vi "PWMControl.vi"() -> ()   [LabVIEW 2016]
uses:
  <vilib>/Utility/error.llb/DialogType.ctl
  <vilib>/DAQmx/write.llb/DAQmx Write (Digital 1D Bool 1Chan 1Samp).vi
  <vilib>/DAQmx/read.llb/DAQmx Read (Analog 1D Wfm NChan NSamp).vi
  <vilib>/DAQmx/configure/task.llb/DAQmx Configure Logging (TDMS).vi
  <vilib>/DAQmx/configure/timing.llb/DAQmx Timing (Sample Clock).vi
  <vilib>/DAQmx/create/channels.llb/DAQmx Create Channel (DO-Digital Output).vi
  <vilib>/DAQmx/miscellaneous.llb/DAQmx Fill In Error Info.vi
  <resource>/objmgr/daqmx.rc
panel:
  in  "Lines":tag="Dev1/port0/line0:7" caption="Digital output line"
  in  "Idle State 2":bool
  in  "Duty cycle % (0-100) 2":dbl=50.0
  in  "Cycle time PWM (seconds) 2":i32=5
  in  "Steps in a cycle 2":i32=256
  out "Output 2":i16(graph)
  in  "base path":path=path "C:/Users/mmunoz/Desktop/Summer Coding Files/Labview Practice Codes/Compiled Data files"
  out "error out":errorcluster
  in  "error in":errorcluster
  in  "Show Configure Dialog?":bool
  in  "Remove Extra Properties? (T)":bool=TRUE
  in  "File Name":string="junk"
  in  "stop 2":bool
  out "Time Elapsed":dbl format="%<%H:%M:%S%2u>t"
  out "Waveform Chart":waveform(dbl)[](graph)
  out "DAQ error":string
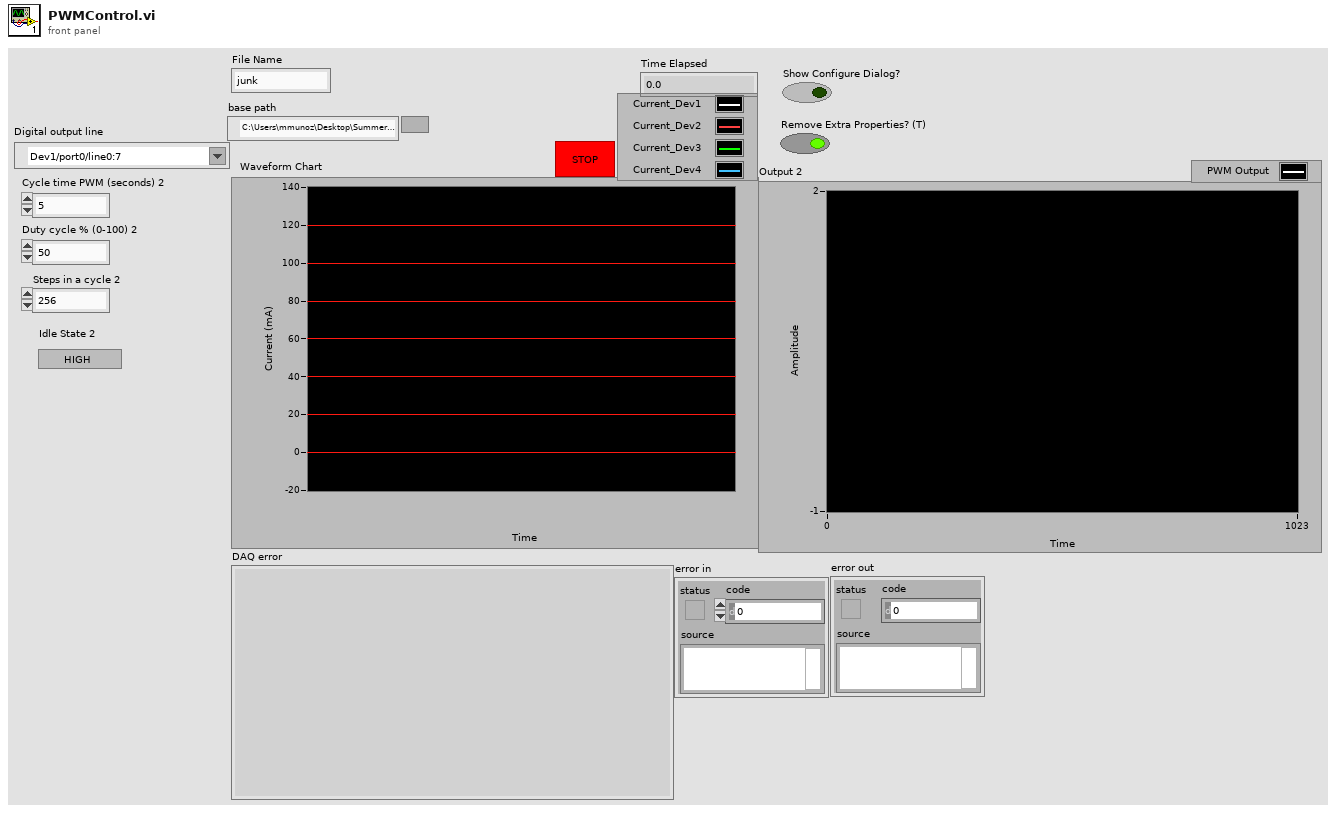
[diagram p1: front panel]
types:
  T1 = typedef "DialogType.ctl" = u16
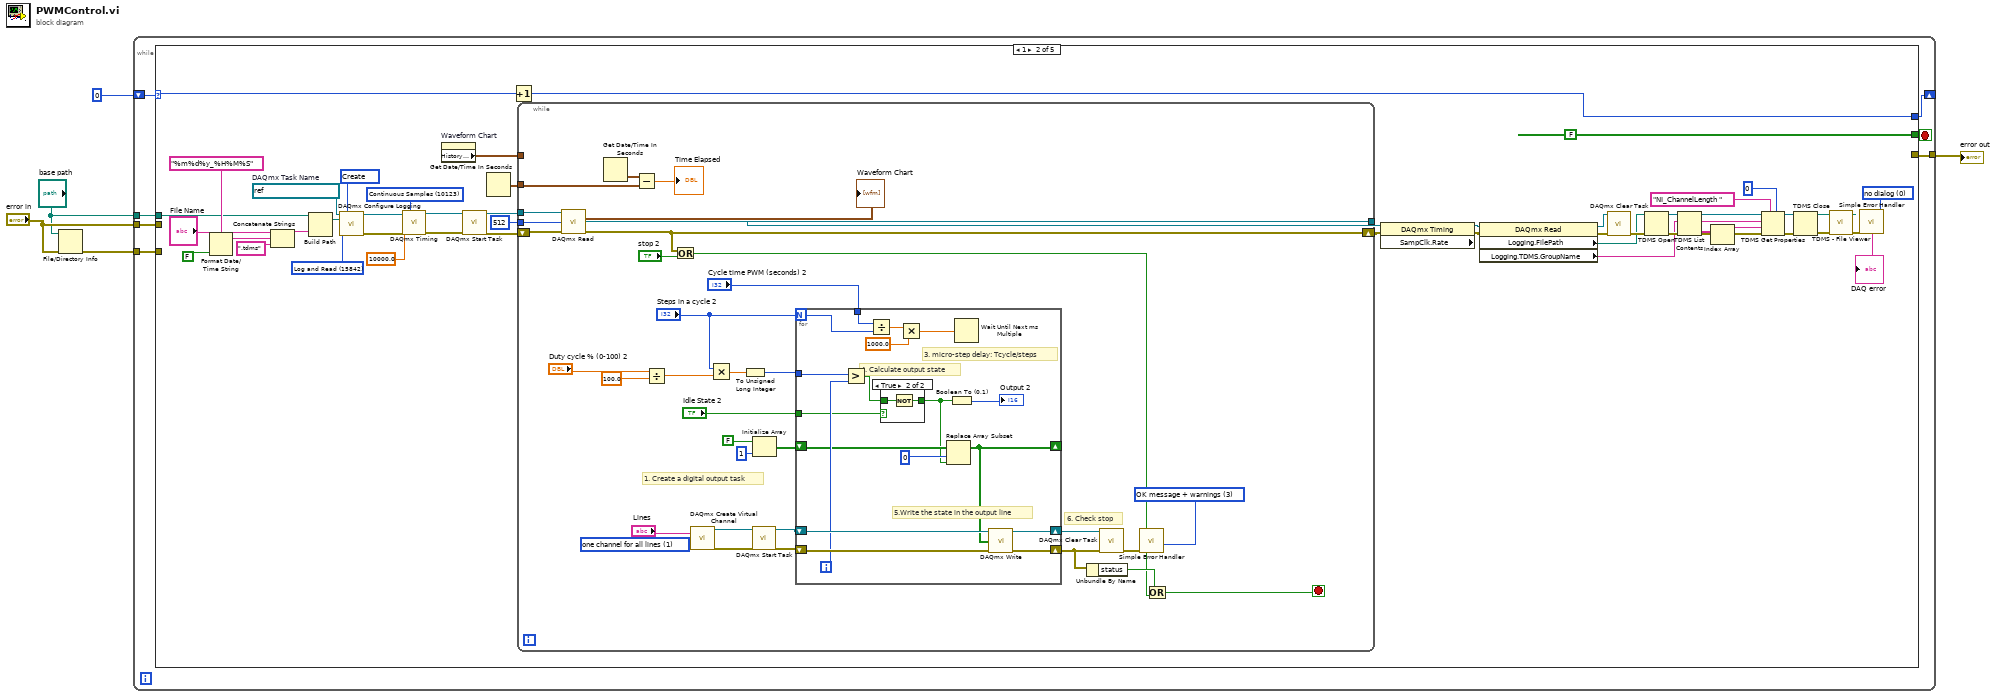
[diagram p0: block diagram]
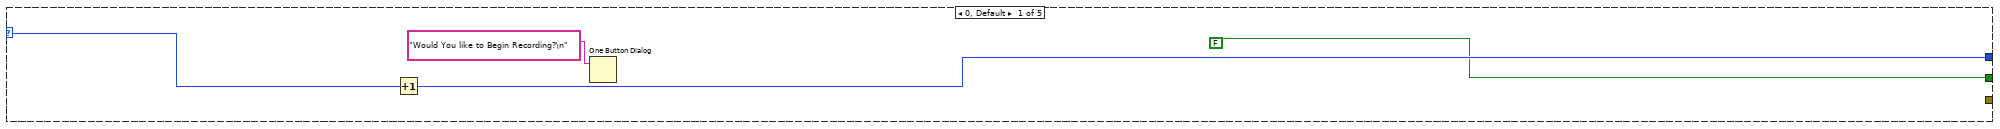
[diagram p2: hidden frame]
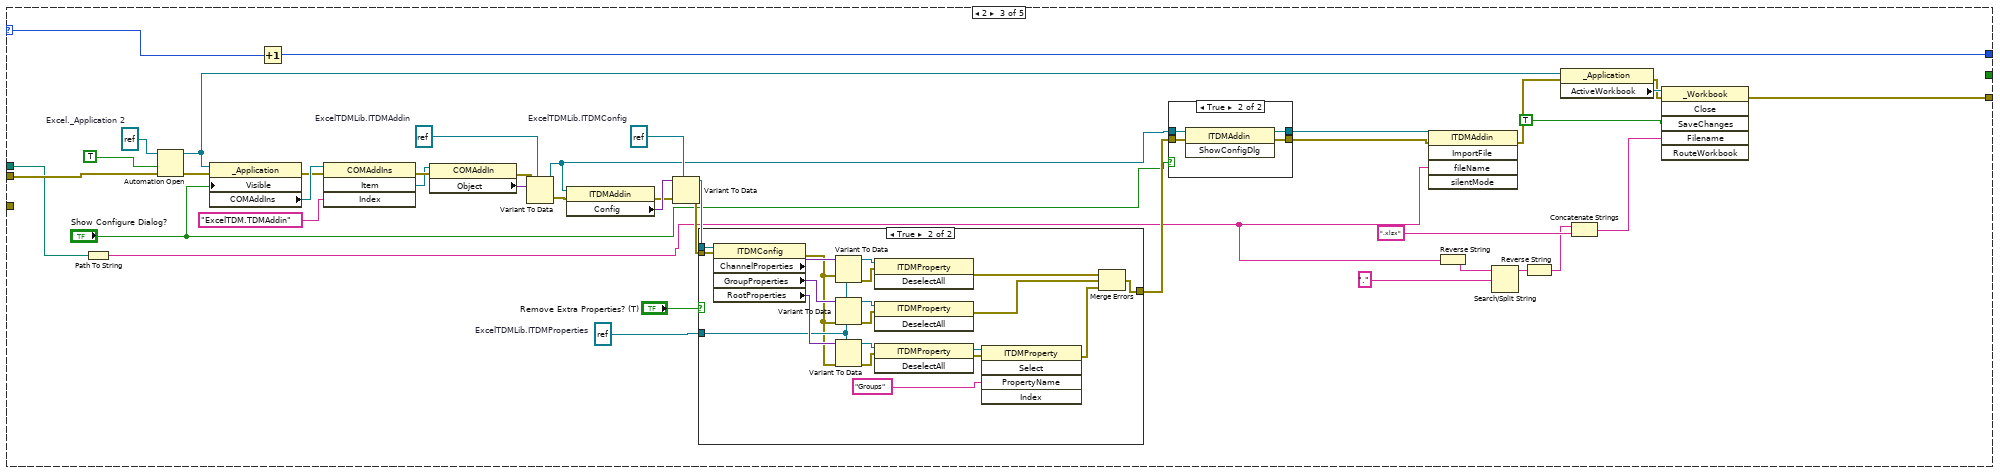
[diagram p4: hidden frame]
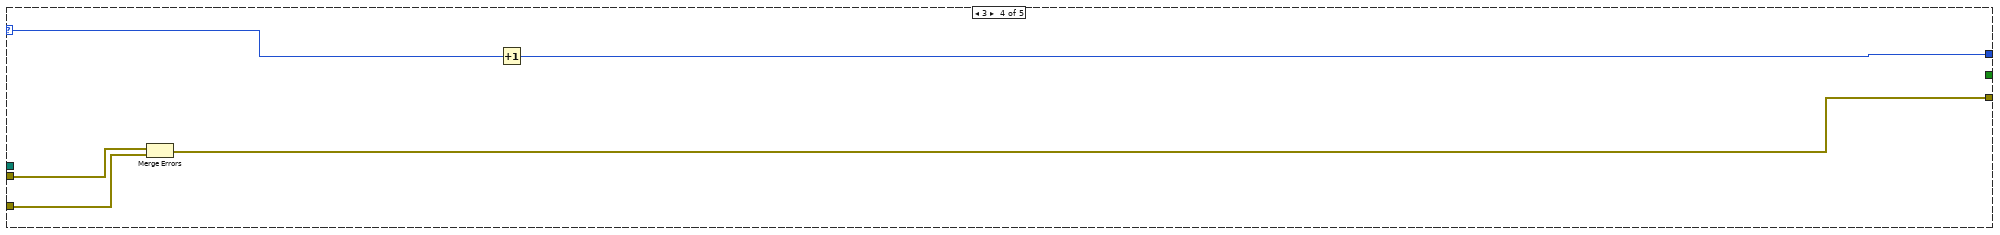
[diagram p7: hidden frame]
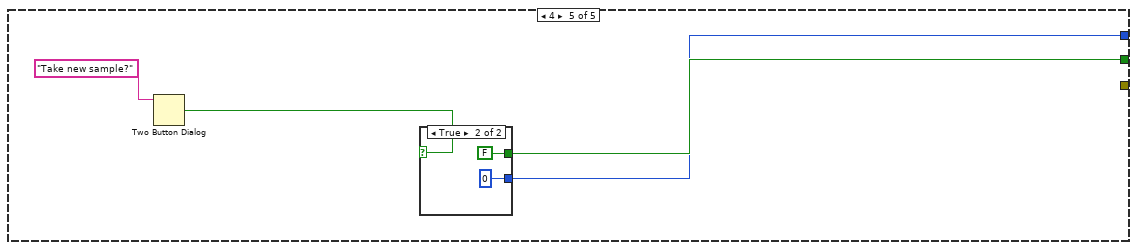
[diagram p8: hidden frame]
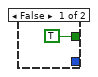
[diagram p9: hidden frame]
diagram:
  n1 = File/Directory Info(path="base path", error in="error in") -> (error out=w3:errorcluster)  [unwired: 6 out]
  n2 = while {
    shift-right: [w11] -> _
    shift-left: 0 -> [w12]
    tunnel: "error in" -> [w10]
    tunnel: w3 -> [w9]
    tunnel: [w8] -> w2
    tunnel: "base path" -> [w7]
    stop <- w6 stop-if-true
    n3 = case shown="1" w12 {
      selector: w12 -> [w13 w44 w162 w191 _]
      tunnel: [w15 w43 w161 w190 w195] -> w11
      tunnel: [FALSE FALSE _ _ w196] -> w6
      tunnel: w10 -> [_ _ w149 w193 _]
      tunnel: w9 -> [_ _ _ w194 _]
      tunnel: [_ _ w128 w192 _] -> w8
      tunnel: w7 -> [_ w17 w122 _ _]
      frame 0, Default {
        n4 = Increment(x=w13) -> (x+1=w15:i32)
        n5 = One Button Dialog(message="Would You like to Begin Recording?\n" ("initial string")) -> ()  [unwired: 1 in, 1 out]
      }
      frame 1 {
        w25 = 10123 items=["Finite Samples"=10178, "Continuous Samples"=10123, "Hardware Timed Single Point"=12522] ("sample mode")
        w52 = T1 0 items=["no dialog", "OK message", "continue or stop message", "OK message + warnings", "continue/stop + warnings"] ("type of dialog (OK msg:1)")
        w57 = 15848 items=["Open"=10437, "Open or Create"=15846, "Create or Replace"=15847, "Create"=15848] ("operation")
        w59 = 15842 items=["Off"=10231, "Log"=15844, "Log and Read"=15842] ("logging mode")
        w60 = refnum<k21> "DAQ Assistant_0"  # DAQmx Task Name
        n6 = Format Date/Time String(time format string (%c)="%m%d%y_%H%M%S", UTC format=FALSE) -> (date/time string=w63:string)  [unwired: 1 in]
        n7 = Concatenate Strings("File Name", w63, ".tdms") -> (w64:string)
        n8 = Build Path(base path=w17, name or relative path=w64) -> (appended path=w58:path)
        n9 = call-poly <vilib>:"DAQmx Configure Logging.vi"("task/channels in"=w60, "operation"=w57, "file path"=w58, "logging mode"=w59) -> ("task out"=w26:refnum<k21>, "error out"=w27:errorcluster)  [unwired: 10 in]
        n10 = call-poly <vilib>:"DAQmx Timing.vi"("task/channels in"=w26, "sample mode"=w25, "rate"=10000.0, "error in"=w27) -> ("task out"=w24:refnum<k21>, "error out"=w23:errorcluster)  [unwired: 10 in]
        n11 = property on="Waveform Chart" class="WFChart (strict)"() -> ("History Data"=w21:waveform(dbl)[][])  [unwired: 2 in, 2 out]
        n12 = call <vilib>:"DAQmx Start Task.vi"("task/channels in"=w24, "error in"=w23) -> ("task out"=w55:refnum<k21>, "error out"=w56:errorcluster)  [unwired: 12 in]
        n13 = Get Date/Time In Seconds() -> (seconds since 1Jan1904=w42:timestamp)
        n14 = Increment(x=w44) -> (x+1=w43:i32)
        n15 = while {
          tunnel: [w99] -> w31
          shift-right: [w92] -> w30
          shift-left: w56 -> [w98]
          tunnel: 512 -> [w97]
          tunnel: w55 -> [w96]
          tunnel: w42 -> [w95]
          tunnel: w21 -> [_]
          stop <- w67 stop-if-true
          w72 = T1 3 items=["no dialog", "OK message", "continue or stop message", "OK message + warnings", "continue/stop + warnings"] ("type of dialog (OK msg:1)")
          w78 = 1 items=["one channel for each line", "one channel for all lines"] ("line grouping")
          # "1. Create a digital output task"
          # "6. Check stop"
          n16 = call-poly <vilib>:"DAQmx Read.vi"("task/channels in"=w96, "number of samples per channel"=w97, "error in"=w98) -> ("task out"=w99:refnum<k21>, "data"=→"Waveform Chart":waveform(dbl)[], "error out"=w92:errorcluster)  [unwired: 10 in]
          n17 = Get Date/Time In Seconds() -> (seconds since 1Jan1904=w94:timestamp)
          n18 = Subtract(x=w94, y=w95) -> (x-y=→"Time Elapsed":dbl)
          n19 = Divide(x="Duty cycle % (0-100) 2", y=100.0) -> (x/y=w87:dbl)
          n20 = Or(x=w92, y="stop 2") -> (x .or. y?=w68:bool)
          n21 = call-poly <vilib>:"DAQmx Create Virtual Channel.vi"("lines"="Lines", "line grouping"=w78) -> ("task out"=w75:refnum<k21>, "error out"=w76:errorcluster)  [unwired: 12 in]
          n22 = Multiply(x="Steps in a cycle 2", y=w87) -> (x*y=w82:dbl)
          n23 = To Unsigned Long Integer(number=w82) -> (unsigned 32bit integer=w81:u32)
          n24 = call <vilib>:"DAQmx Start Task.vi"("task/channels in"=w75, "error in"=w76) -> ("task out"=w74:refnum<k21>, "error out"=w73:errorcluster)  [unwired: 12 in]
          n25 = Initialize Array(FALSE, 1 ("dimension size")) -> (w84:bool[])
          n26 = for {
            N: "Steps in a cycle 2" -> [w117]
            tunnel: "Cycle time PWM (seconds) 2" -> [w118]
            tunnel: w81 -> [w114]
            shift-right: [w113] -> w71
            shift-left: w74 -> [w110]
            shift-right: [w112] -> w70
            shift-left: w73 -> [w111]
            shift-right: [w105] -> _
            shift-left: w84 -> [w106]
            tunnel: "Idle State 2" -> [w104]
            i -> [w107]
            # "5.Write the state in the output line"
            # "4. Calculate output state"
            # "3. micro-step delay: Tcycle/steps"
            n27 = Greater?(x=w114, y=w107) -> (0:w103:bool)
            n28 = Divide(x=w118, y=w117) -> (x/y=w116:dbl)
            n29 = case shown="True" w104 {
              tunnel: [w119 w120] -> w102
              tunnel: w103 -> [w119 w121]
              frame False {
              }
              frame True {
                n30 = Not(x=w121) -> (.not. x?=w120:bool)
              }
            }
            n31 = Multiply(x=w116, y=1000.0) -> (x*y=w109:dbl)
            n32 = Replace Array Subset(array=w106, new element=w102, index=0) -> (w105:bool[])
            n33 = Boolean To (0,1)(Boolean=w102) -> (0, 1=→"Output 2":i16)
            n34 = Wait Until Next ms Multiple(millisecond multiple=w109) -> ()  [unwired: 1 out]
            n35 = call-poly <vilib>:"DAQmx Write.vi"("task/channels in"=w110, "data"=w105, "error in"=w111) -> ("task out"=w113:refnum<k21>, "error out"=w112:errorcluster)  [unwired: 10 in, 1 out]
          }
          n36 = Unbundle By Name(w70) -> ("status"=w79:bool)
          n37 = call <vilib>:"DAQmx Clear Task.vi"("task in"=w71, "error in"=w70) -> ("error out"=w69:errorcluster)  [unwired: 13 in]
          n38 = call <vilib>:"Simple Error Handler.vi"("type of dialog (OK msg:1)"=w72, "error in (no error)"=w69) -> ()  [unwired: 3 in, 5 out]
          n39 = Or(x=w79, y=w68) -> (x .or. y?=w67:bool)
        }
        n40 = property on="Property Node" class="DAQmx Timing" props=["SampClk.Rate"](reference=w31, error in=w30) -> (reference out=w29:refnum<k21>, error out=w28:errorcluster)  [unwired: 1 out]
        n41 = property on="Property Node" class="DAQmx Read"(reference=w29, error in=w28) -> (reference out=w51:refnum<k21>, error out=w50:errorcluster, "Logging.FilePath"=w45:path, "Logging.TDMS.GroupName"=w39:string)
        n42 = call <vilib>:"DAQmx Clear Task.vi"("task in"=w51, "error in"=w50) -> ("error out"=w46:errorcluster)  [unwired: 13 in]
        n43 = TDMS Open(8:w46, 11:w45) -> (0:w40:errorcluster, 3:w38:refnum<k34>)  [unwired: 5 in]
        n44 = TDMS List Contents(4:w40, 6:w39, 7:w38) -> (0:w18:errorcluster, 1:w36:string[], 2:w37:string, 3:w33:refnum<k34>)
        n45 = Index Array(array=w36) -> (element=w35:string)  [unwired: 1 in]
        n46 = TDMS Get Properties(5:0, 7:"NI_ChannelLength " ("property name"), 8:w18, 9:w35, 10:w37, 11:w33) -> (0:w19:errorcluster, 3:w20:refnum<k34>)  [unwired: 4 out]
        n47 = TDMS Close(8:w19, 11:w20) -> (0:w48:errorcluster, 3:w47:path)
        n48 = call <vilib>:"TDMS - File Viewer.vi"("error in (no error)"=w48, "file path"=w47) -> ("error out"=w49:errorcluster)  [unwired: 4 in, 1 out]
        n49 = call <vilib>:"Simple Error Handler.vi"("error code (no error:0)"=w52, "error in (no error)"=w49) -> ("message"=→"DAQ error":string)  [unwired: 3 in, 4 out]
      }
      frame 2 {
        w147 = refnum<k7> refnum  # ExcelTDMLib.ITDMProperties
        w158 = refnum<k7> refnum  # Excel._Application 2
        w154 = refnum<k7> refnum  # ExcelTDMLib.ITDMConfig
        w159 = refnum<k7> refnum  # ExcelTDMLib.ITDMAddin
        n50 = Path To String(path=w122) -> (string=w129:string)
        n51 = Automation Open(error in (no error)=w149, Automation Refnum=w158, 9:TRUE ("open new instance (false)")) -> (Automation Refnum=w127:refnum<k7>, error out=w157:errorcluster)  [unwired: 1 in]
        n52 = property class="_Application"(reference=w127, error in=w157, "Visible"="Show Configure Dialog?") -> (error out=w155:errorcluster, "COMAddIns"=w160:refnum<k7>)  [unwired: 1 out]
        n53 = Increment(x=w162) -> (x+1=w161:i32)
        n54 = invoke class="COMAddIns" method="Item"(reference=w160, error in=w155, "Index"="ExcelTDM.TDMAddin") -> (error out=w126:errorcluster, "Item"=w125:refnum<k7>)  [unwired: 1 in, 2 out]
        n55 = property class="COMAddIn"(reference=w125, error in=w126) -> (error out=w123:errorcluster, "Object"=w124:variant)  [unwired: 1 out]
        n56 = Variant To Data(error in=w123, type=w159, Variant=w124) -> (data=w143:refnum<k7>, error out=w152:errorcluster)
        n57 = property class="ITDMAddin"(reference=w143, error in=w152) -> (error out=w151:errorcluster, "Config"=w153:variant)  [unwired: 1 out]
        n58 = Variant To Data(error in=w151, type=w154, Variant=w153) -> (data=w144:refnum<k7>, error out=w145:errorcluster)
        n59 = case shown="True" "Remove Extra Properties? (T)" {
          tunnel: w147 -> [_ w185]
          tunnel: w145 -> [w169 w176]
          tunnel: w144 -> [_ w175]
          tunnel: [w169 w174] -> w146
          frame False {
          }
          frame True {
            n60 = property class="ITDMConfig"(reference=w175, error in=w176) -> (error out=w180:errorcluster, "ChannelProperties"=w189:variant, "GroupProperties"=w187:variant, "RootProperties"=w186:variant)  [unwired: 1 out]
            n61 = Variant To Data(error in=w180, type=w185, Variant=w189) -> (data=w188:refnum<k7>, error out=w177:errorcluster)
            n62 = Variant To Data(error in=w180, type=w185, Variant=w187) -> (data=w183:refnum<k7>, error out=w178:errorcluster)
            n63 = Variant To Data(error in=w180, type=w185, Variant=w186) -> (data=w184:refnum<k7>, error out=w179:errorcluster)
            n64 = invoke class="ITDMProperty" method="DeselectAll"(reference=w188, error in=w177) -> (error out=w181:errorcluster)  [unwired: 1 in, 2 out]
            n65 = invoke class="ITDMProperty" method="DeselectAll"(reference=w183, error in=w178) -> (error out=w182:errorcluster)  [unwired: 1 in, 2 out]
            n66 = invoke class="ITDMProperty" method="DeselectAll"(reference=w184, error in=w179) -> (reference out=w173:refnum<k7>, error out=w172:errorcluster)  [unwired: 1 in, 1 out]
            n67 = invoke class="ITDMProperty" method="Select"(reference=w173, error in=w172, "PropertyName"="Groups" ("string")) -> (error out=w171:errorcluster)  [unwired: 2 in, 4 out]
            n68 = Merge Errors(w181, w182, w171) -> (w174:errorcluster)
          }
        }
        n69 = case shown="True" "Show Configure Dialog?" {
          tunnel: w143 -> [w164 w168]
          tunnel: w146 -> [w163 w167]
          tunnel: [w163 w166] -> w130
          tunnel: [w164 w165] -> w131
          frame False {
          }
          frame True {
            n70 = invoke class="ITDMAddin" method="ShowConfigDlg"(reference=w168, error in=w167) -> (reference out=w165:refnum<k7>, error out=w166:errorcluster)  [unwired: 1 in, 1 out]
          }
        }
        n71 = invoke class="ITDMAddin" method="ImportFile"(reference=w131, error in=w130, "fileName"=w129) -> (error out=w141:errorcluster)  [unwired: 2 in, 4 out]
        n72 = Reverse String(1:w129) -> (0:w135:string)
        n73 = Search/Split String(string=w135, search string/char (-)=".") -> (substring before match=w133:string)  [unwired: 1 in, 2 out]
        n74 = Reverse String(1:w133) -> (0:w132:string)
        n75 = property class="_Application"(reference=w127, error in=w141) -> (error out=w136:errorcluster, "ActiveWorkbook"=w140:refnum<k7>)  [unwired: 1 out]
        n76 = Concatenate Strings(w132, ".xlsx" ("string")) -> (w137:string)
        n77 = invoke class="_Workbook" method="Close"(reference=w140, error in=w136, "SaveChanges"=TRUE, "Filename"=w137) -> (error out=w128:errorcluster)  [unwired: 2 in, 5 out]
      }
      frame 3 {
        n78 = Merge Errors(w193, w194) -> (w192:errorcluster)
        n79 = Increment(x=w191) -> (x+1=w190:i32)
      }
      frame 4 {
        n80 = Two Button Dialog(message="Take new sample?") -> (T button?=w197:bool)  [unwired: 2 in]
        n81 = case shown="True" w197 {
          tunnel: [TRUE FALSE] -> w196
          tunnel: [_ 0] -> w195
          frame False {
          }
          frame True {
          }
        }
      }
    }
  }
  "error out" <- w2
